vi "2ndStrikerNormalV1.vi"(4 "Impulso de\ntime elapsed":bool=TRUE, 5 "Stop":bool, 6 "atacando ao contrário?":bool=TRUE, 7 "AI Parameters":T1={"GotoKick"={"Dist do cone a frente"=150.0, "attacker farback"=1500.0, "Perto"=300.0, "min dist to kick"=150.0, "kick eps"=0.0, "Time to transition"=0.05}, "Attacker"={"CC chute"=0.09, "CC passe"=0.045, "Kick Force"=100.0, "ball-robot Kick"=200.0, "ball-robot Pass"=0.3, "drible\nAttk"=FALSE}, "Defender"={"D max"=1700.0, "Vel p/ robô av"=1000.0, "Kick Force"=100.0, "D atk-def"=0.0, "D farback"=0.0, "drible\ndef"=FALSE, "drible\ngoalie"=FALSE}, "Timeout"={"Field/v in x"=6.0, "Dist Robots"=300, "Dist up in y"=300}, "Pose Striker"={"dist"=200.0, "Numeric"=-4.0, "dist 2"=200.0, "drible\nstriker"=FALSE}, "Dist Stop"=300.0, "D ball out"=200, "D central gap "=150.0, "T pass"=0.0, "Force ++"=0.0, "range kick"=0.0, "Chute alto"=TRUE, "Marcador novo"=TRUE, "drible"=FALSE, "D drible"=300.0, "Versão Striker"=enum."3", "Defesa"=enum."ManMark", "Marcador"=enum."Marcar Segndo mais perigoso", "Receptor passe"=enum."2nd Striker"} {"D drible" format="%#_13g"; "D central gap" format="%#_13g"; "Dist Stop" format="%#_13g"; "Pose Striker"."Numeric" format="%#_13g"; "Defender"."Kick Force" format="%#_13g"; "Defender"."Vel p/ robô av" format="%#_13g"; "Attacker"."ball-robot Kick" format="%#_13g"; "Attacker"."Kick Force" format="%#_13g"; "Attacker"."CC passe" format="%#_13g"; "Attacker"."CC chute" format="%#_13g"; "GotoKick"."kick eps" format="%#_13g"; "GotoKick"."min dist to kick" format="%#_13g"; "GotoKick"."Perto" format="%#_13g"; "GotoKick"."attacker farback" format="%#_13g"; "GotoKick"."Dist do cone a frente" format="%#_13g"}, 8 "IA Input":T9={"our_robots"=[], "enemy_robots"=[], "balls"=[], "geometry"={"line_width"=0, "field_length"=0, "field_width"=0, "boundary_width"=0, "referee_width"=0, "goal_width"=0, "goal_depth"=0, "goal_wall_width"=0, "center_circle_radius"=0, "defense_radius"=0, "defense_stretch"=0, "free_kick_from_defense_dist"=0, "penalty_spot_from_field_line_dist"=0, "penalty_line_from_spot_dist"=0}, "IA Judge"={"stage"="", "command"="", "our_goalie_id"=0.0, "enemy_goalie_id"=0.0, "command enum"=enum."Halt", "Time"=enum."Azul"}, "Received Timestamp"=timestamp(0 s since 1904-01-01), "Events"={"Touch"=FALSE, "Ball out"=FALSE, "id touch"=0.0, "Ball out of \nVision"=FALSE, "Ball inside \nGoalie area"=FALSE, "Robot not responding"=FALSE, "Robots responding status"=[1.0, 1.0, 1.0, 1.0, 1.0, 1.0], "Enemy Ball \nPossession"=FALSE, "Pass State"=FALSE, "id end of pass"=0.0, "Kick"=FALSE, "Id ini Possession"=0.0, "Ball Possesion"=FALSE, "Id Possesion"=0.0, "Direct Kick"=FALSE, "2nd Strk Ativo"=FALSE}}, 9 "balls":T7[](array[typedef])=[{"x"=-2165.869384765625, "y"=510.4085693359375, "timestamp"=timestamp(2082758857.4639893 s since 1904-01-01), "Vel_x"=0.0, "Vel_y"=0.0, "Pos Bola Est"=[]}], 10 "Field Size in":T8={"line_width"=10, "field_length"=6000, "field_width"=4000, "boundary_width"=250, "referee_width"=425, "goal_width"=700, "goal_depth"=180, "goal_wall_width"=20, "center_circle_radius"=500, "defense_radius"=500, "defense_stretch"=350, "free_kick_from_defense_dist"=700, "penalty_spot_from_field_line_dist"=450, "penalty_line_from_spot_dist"=350}, 11 "Robot in":T2={"id"=5, "function"=enum."Attacker", "x"=-1842.5054931640625, "y"=520.60986328125, "orientation"=-2.7555055618286133, "v_tangent"=0.0, "v_normal"=0.0, "v_ang"=0.0, "kick_x"=0.0, "kick_z"=0.0, "dribble"=FALSE, "Timestamp"=timestamp(2082758857.4639893 s since 1904-01-01), "estimatives"={"est_v_tangent"=0.0, "est_v_normal"=0.0, "est_vx"=0.0, "est_vy"=0.0, "Pos Robot Est"=[]}, "dest_x_kick"=0.0, "dest_y_kick"=0.0, "Gap Coord"=[], "States"=enum."GoToTangent", "Path "=[], "Path  Smooth"=[], "Dest"=[]}) -> (2 "Robot out":T2={"id"=5, "function"=enum."Attacker", "x"=-1842.5054931640625, "y"=520.60986328125, "orientation"=-2.7555055618286133, "v_tangent"=-0.08361641967936218, "v_normal"=-0.20513016702014014, "v_ang"=0.24456003022714357, "kick_x"=0.0, "kick_z"=0.0, "dribble"=FALSE, "Timestamp"=timestamp(2082758857.4639893 s since 1904-01-01), "estimatives"={"est_v_tangent"=0.0, "est_v_normal"=0.0, "est_vx"=0.0, "est_vy"=0.0, "Pos Robot Est"=[]}, "dest_x_kick"=0.0, "dest_y_kick"=0.0, "Gap Coord"=[], "States"=enum."GoToTangent", "Path "=[], "Path  Smooth"=[], "Dest"=[]})   [LabVIEW 2017]
uses:
  Core/AI Robot.ctl
  Functions Enum.ctl
  AttackerStates.ctl
  Path Planning/RRT/PathDests.ctl
  Path Planning/RRT/PathDest.ctl
  Core/AI Input.ctl
  Core/AI Ball.ctl
  Core/Field Size.ctl
  Core/AI Judge.ctl
  Command Enum.ctl
  Util/Events/Events.ctl
  AI Parameters.ctl
panel:
  in  "Wait pass perpendicular?":bool=TRUE
  in  "Marcador sempre":bool
  out "size(s)":i32
  in  "IDattacker":dbl
  in  "Yattacker":dbl
  in  "Xattacker":dbl
  out "States":T4
  out "sentido":dbl
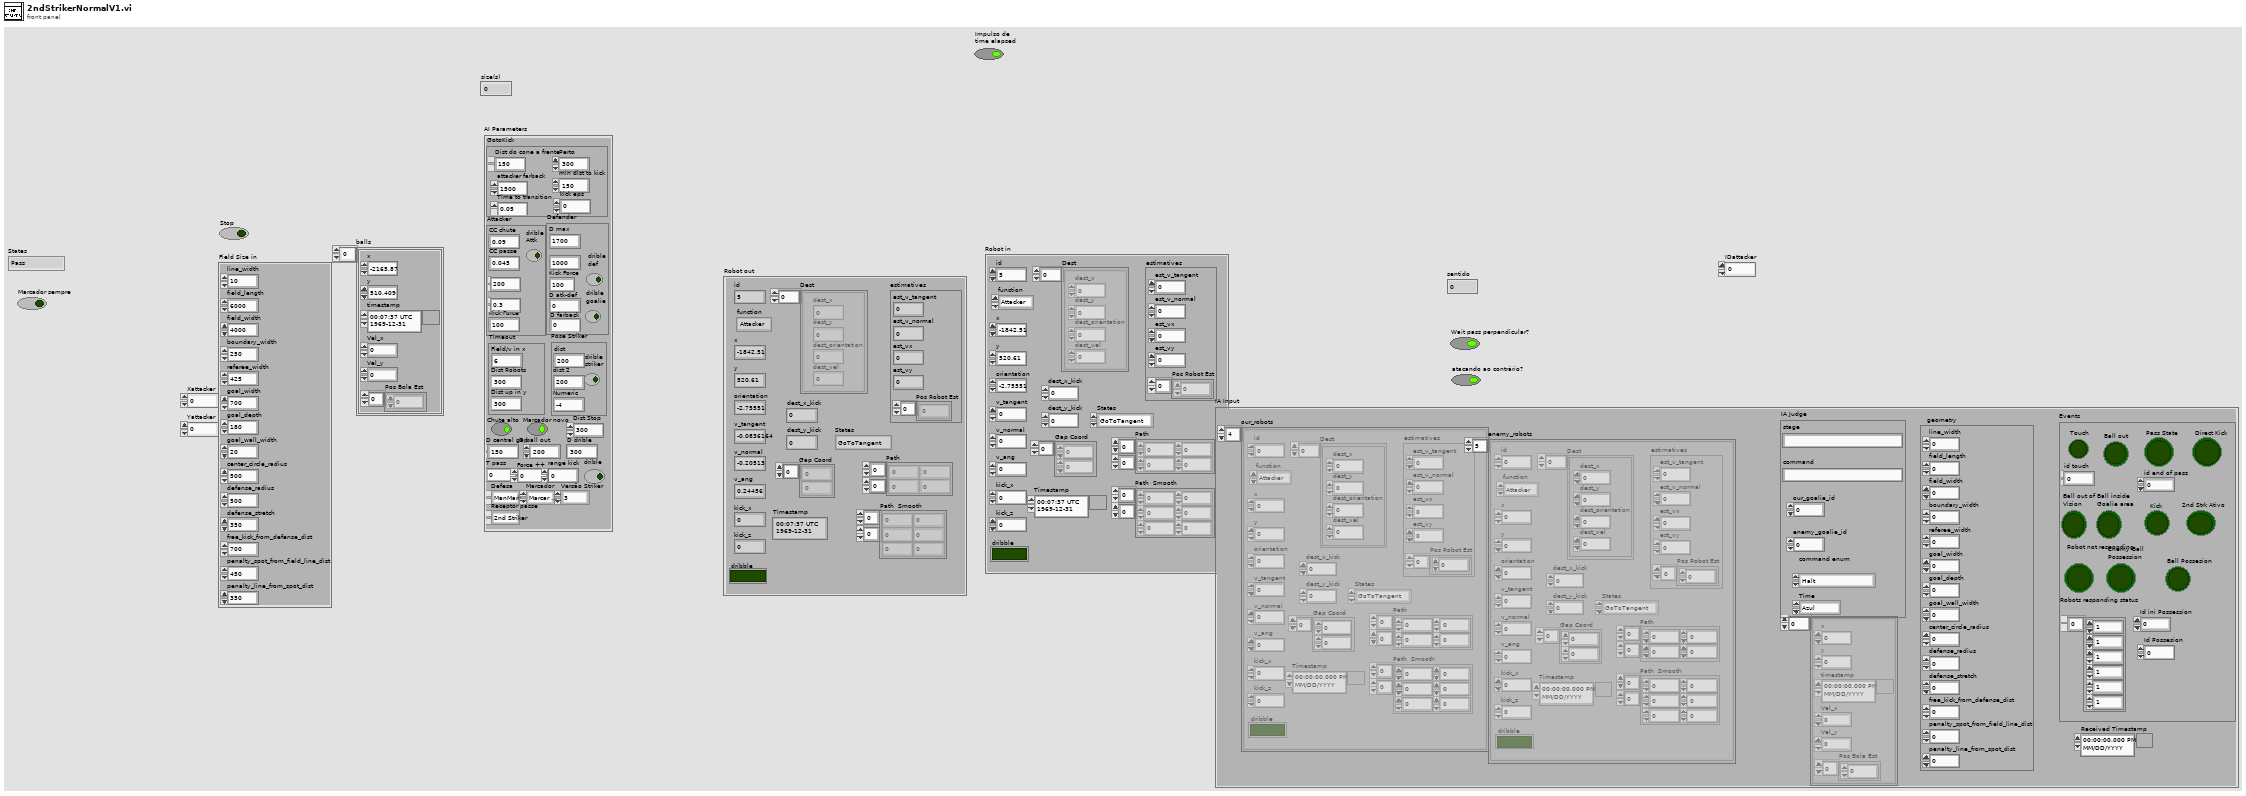
[diagram p1: front panel]
types:
  T1 = typedef "AI Parameters.ctl" = cluster{"GotoKick":cluster{"Dist do cone a frente":dbl, "attacker farback":dbl, "Perto":dbl, "min dist to kick":dbl, "kick eps":dbl, "Time to transition":dbl}, "Attacker":cluster{"CC chute":dbl, "CC passe":dbl, "Kick Force":dbl, "ball-robot Kick":dbl, "ball-robot Pass":dbl, "drible\nAttk":bool}, "Defender":cluster{"D max":dbl, "Vel p/ robô av":dbl, "Kick Force":dbl, "D atk-def":dbl, "D farback":dbl, "drible\ndef":bool, "drible\ngoalie":bool}, "Timeout":cluster{"Field/v in x":dbl, "Dist Robots":u32, "Dist up in y":u32}, "Pose Striker":cluster{"dist":dbl, "Numeric":dbl, "dist 2":dbl, "drible\nstriker":bool}, "Dist Stop":dbl, "D ball out":i32, "D central gap ":dbl, "T pass":dbl, "Force ++":dbl, "range kick":dbl, "Chute alto":bool, "Marcador novo":bool, "drible":bool, "D drible":dbl, "Versão Striker":enum16{"3", "2", "1"}, "Defesa":enum16{"ManMark", "Barreira"}, "Marcador":enum16{"Marcar Segndo mais perigoso", "Marcar o mais perigoso"}, "Receptor passe":enum16{"2nd Striker", "Striker"}}
  T2 = typedef "AI Robot.ctl" = cluster{"id":u32, "function":T3, "x":dbl, "y":dbl, "orientation":dbl, "v_tangent":dbl, "v_normal":dbl, "v_ang":dbl, "kick_x":dbl, "kick_z":dbl, "dribble":bool, "Timestamp":timestamp, "estimatives":cluster{"est_v_tangent":dbl, "est_v_normal":dbl, "est_vx":dbl, "est_vy":dbl, "Pos Robot Est":dbl[]}, "dest_x_kick":dbl, "dest_y_kick":dbl, "Gap Coord":dbl[], "States":T4, "Path ":dbl[][], "Path  Smooth":dbl[][], "Dest":T5}
  T3 = typedef "Functions Enum.ctl" = enum16{"2nd Striker", "Attacker", "Goalie", "Defender", "Striker", "Goto 0", "Dummy", "Kicker", "ZigZag 0", "ZigZag 1", "ZigZag 2", "ZigZag 3", "ZigZag 4", "ZigZag 5", "ZigZag 6", "ZigZag 7", "ZigZag 8", ""}
  T4 = typedef "AttackerStates.ctl" = enum16{"Pass", "GoToTangent", "BallGetting", "GoToKick", ""}
  T5 = typedef "PathDests.ctl" = T6[]
  T6 = typedef "PathDest.ctl" = cluster{"dest_x":dbl, "dest_y":dbl, "dest_orientation":dbl, "dest_vel":dbl}
  T7 = typedef "AI Ball.ctl" = cluster{"x":dbl, "y":dbl, "timestamp":timestamp, "Vel_x":dbl, "Vel_y":dbl, "Pos Bola Est":dbl[]}
  T8 = typedef "Field Size.ctl" = cluster{"line_width":u32, "field_length":u32, "field_width":u32, "boundary_width":u32, "referee_width":u32, "goal_width":u32, "goal_depth":u32, "goal_wall_width":u32, "center_circle_radius":u32, "defense_radius":u32, "defense_stretch":u32, "free_kick_from_defense_dist":u32, "penalty_spot_from_field_line_dist":u32, "penalty_line_from_spot_dist":u32}
  T9 = typedef "AI Input.ctl" = cluster{"our_robots":T2[], "enemy_robots":T2[], "balls":T7[], "geometry":T8, "IA Judge":T10, "Received Timestamp":timestamp, "Events":T12}
  T10 = typedef "AI Judge.ctl" = cluster{"stage":string, "command":string, "our_goalie_id":dbl, "enemy_goalie_id":dbl, "command enum":T11, "Time":enum16{"Azul", "Amarelo"}}
  T11 = typedef "Command Enum.ctl" = enum16{"Halt", "Stop", "Force Start", "PKA Normal Start", "Prepare Kickoff Ally", "PKE Normal Start", "Prepare Kickoff Enemy", "Prepare Penalty Ally", "PPA Normal Start", "Prepare Penalty Enemy", "PPE Normal Start", "Direct Free Enemy", "Direct Free Ally", "Indirect Free Enemy", "Indirect Free Ally", "Timeout Enemy", "Timeout Ally", "Goal Enemy", "Goal Ally", "Ball Placement Enemy", "Ball Placement Ally", "Normal Half Time", "Extra Time Break", "Extra Half Time", "None", "Post Game"}
  T12 = typedef "Events.ctl" = cluster{"Touch":bool, "Ball out":bool, "id touch":dbl, "Ball out of \nVision":bool, "Ball inside \nGoalie area":bool, "Robot not responding":bool, "Robots responding status":dbl[], "Enemy Ball \nPossession":bool, "Pass State":bool, "id end of pass":dbl, "Kick":bool, "Id ini Possession":dbl, "Ball Possesion":bool, "Id Possesion":dbl, "Direct Kick":bool, "2nd Strk Ativo":bool}
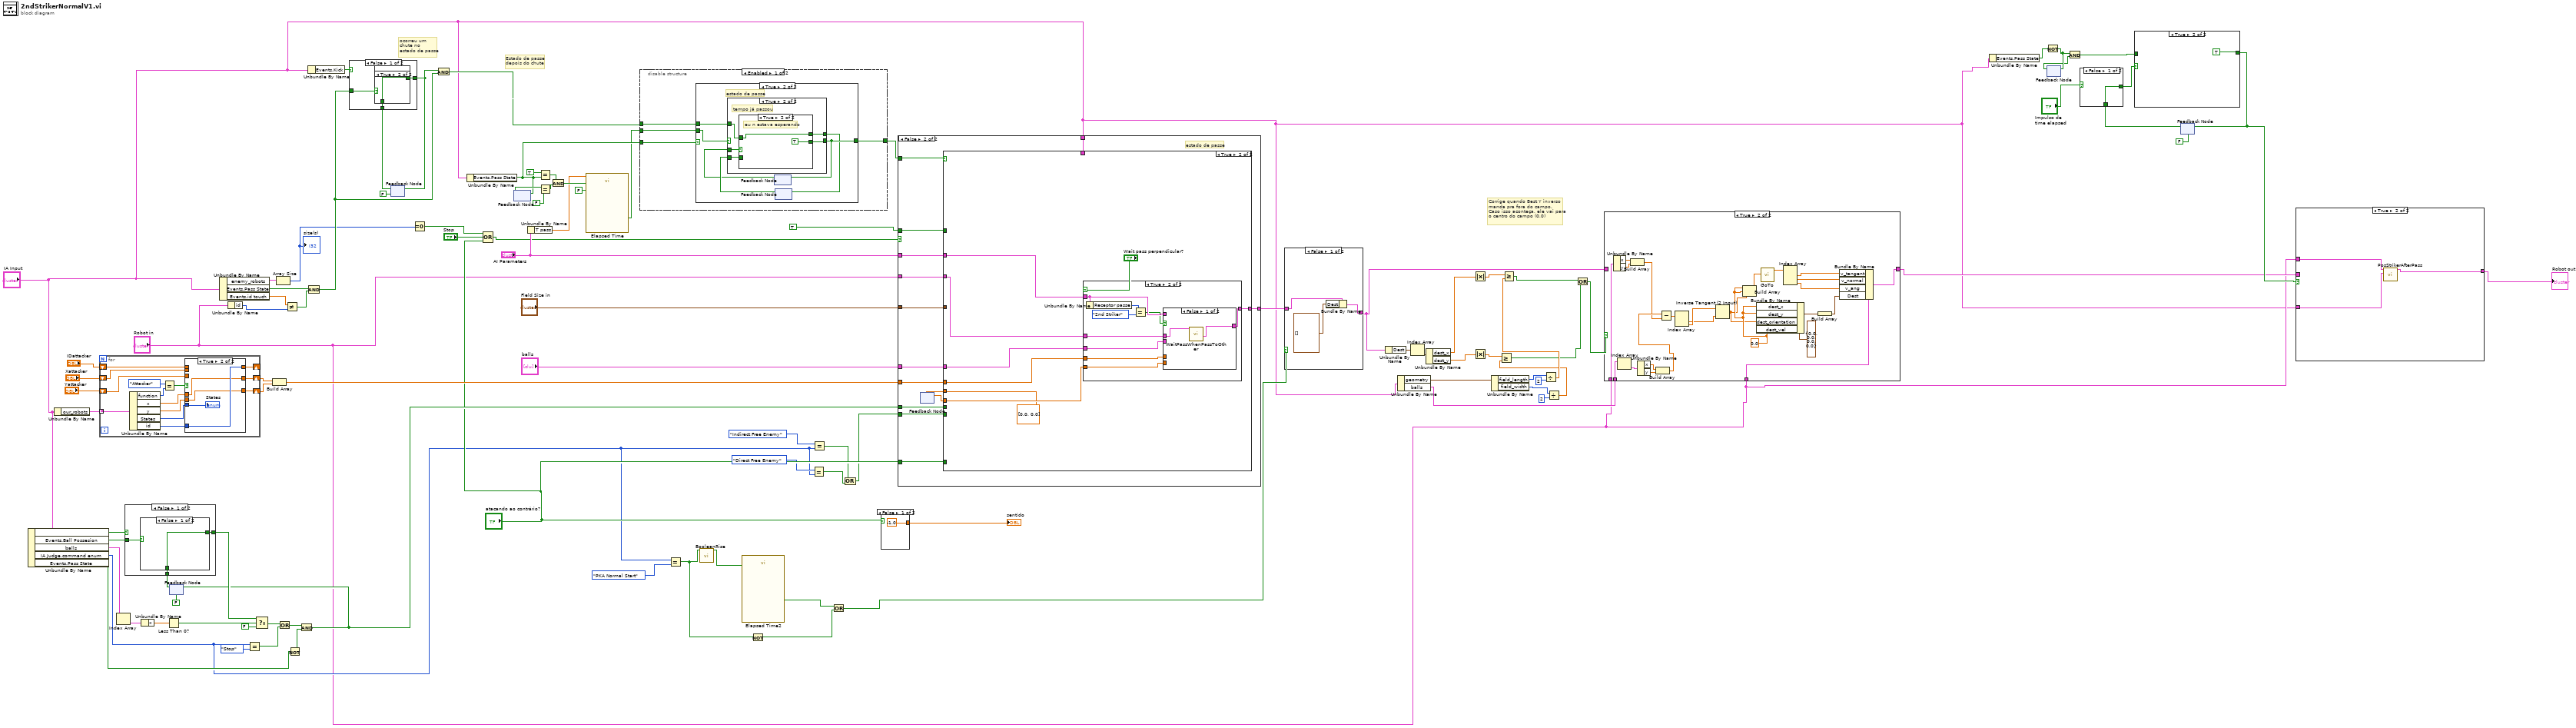
[diagram p0: block diagram]
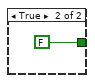
[diagram p2: hidden frame]
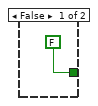
[diagram p7: hidden frame]
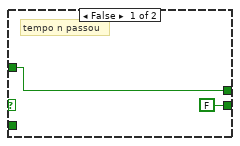
[diagram p8: hidden frame]
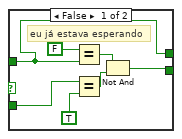
[diagram p9: hidden frame]
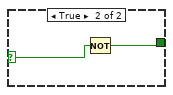
[diagram p11: hidden frame]
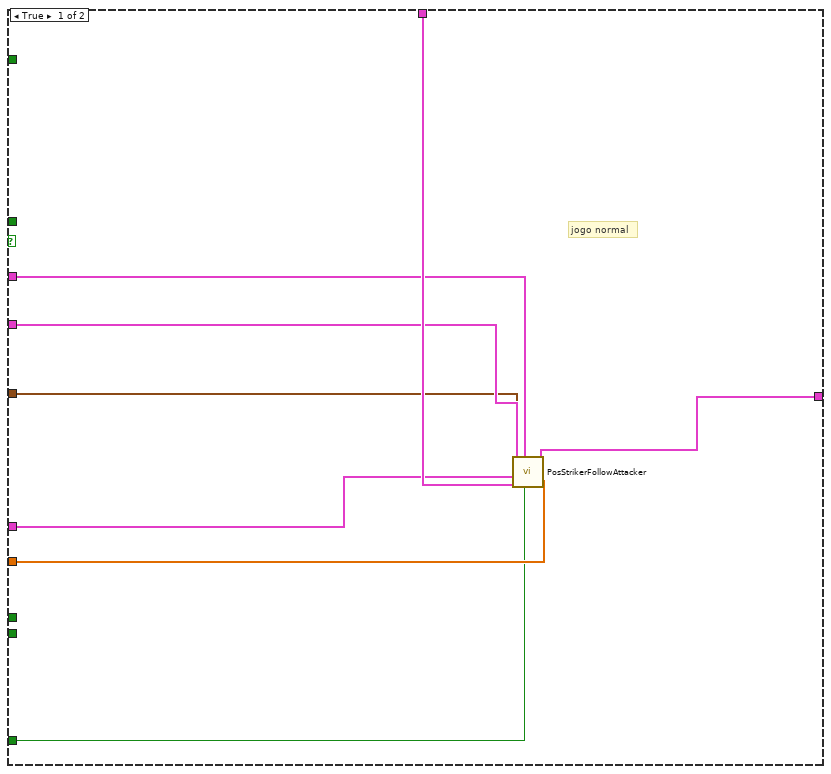
[diagram p13: hidden frame]
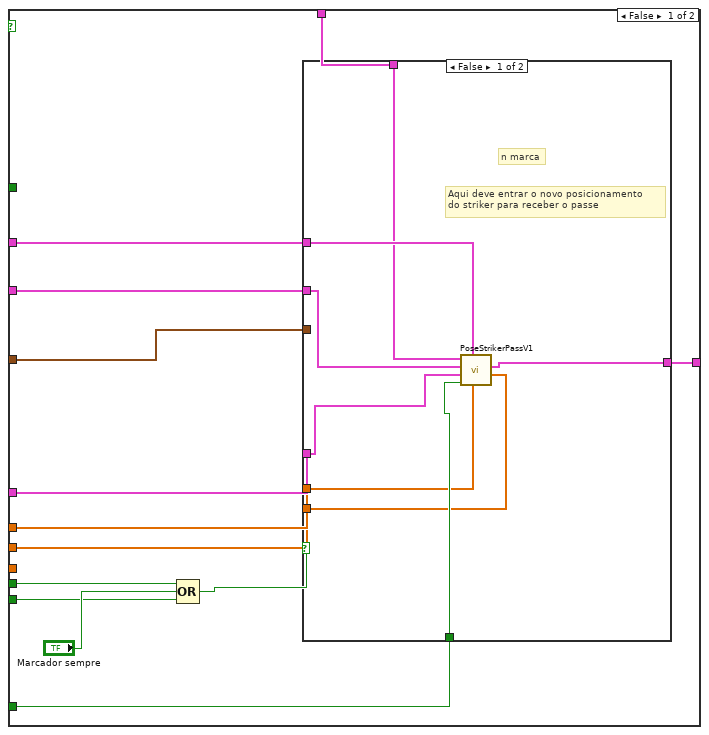
[diagram p14: hidden frame]
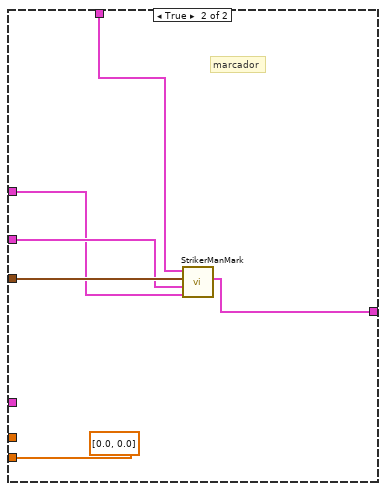
[diagram p15: hidden frame]
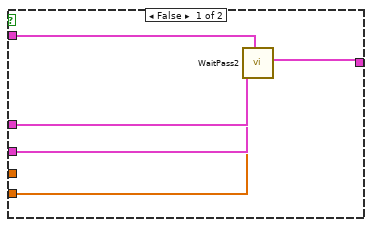
[diagram p16: hidden frame]
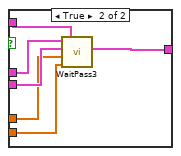
[diagram p17: hidden frame]
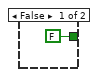
[diagram p19: hidden frame]
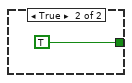
[diagram p20: hidden frame]
diagram:
  # "Corrige quando Best Y inverso\nmanda pra fora do campo.\nCaso isso aconteça, ele vai para\no centro do campo (0,0)"
  # "ocorreu um \nchute no\nestado de passe"
  # "Estado de passe\ndepois do chute"
  n1 = Unbundle By Name("IA Input") -> ("Events.Enemy Ball \nPossession"=w79:bool, "Events.Ball Possesion"=w78:bool, "balls"=w76:T7[], "IA Judge.command enum"=w39:T11, "Events.Pass State"=w66:bool)
  n2 = Unbundle By Name("IA Input") -> ("our_robots"=w94:T2[])
  n3 = for {
    tunnel: w94 -> [w109] mode=indexing
    shift-right: [w105] -> w90
    shift-left: "Xattacker" -> [w103]
    shift-right: [w104] -> w89
    shift-left: "Yattacker" -> [w102]
    shift-right: [w106] -> _
    shift-left: "IDattacker" -> [w101]
    n4 = Unbundle By Name(w109) -> ("function"=w114:T3, "x"=w111:dbl, "y"=w110:dbl, "States"=w108:T4, "id"=w107:u32)
    n5 = Equal?(x=Functions_Enum."Attacker", y=w114) -> (x = y?=w112:bool)
    n6 = case shown="True" w112 {
      tunnel: w111 -> [_ w119]
      tunnel: w110 -> [_ w118]
      tunnel: w108 -> [_ w121]
      tunnel: w107 -> [_ w120]
      tunnel: [w115 w120] -> w106
      tunnel: [w117 w119] -> w105
      tunnel: [w116 w118] -> w104
      tunnel: w103 -> [w117 _]
      tunnel: w102 -> [w116 _]
      tunnel: w101 -> [w115 _]
      frame False {
      }
      frame True {
        "States" <- w121
      }
    }
  }
  n7 = Index Array(array=w76) -> (element=w75:T7)  [unwired: 1 in]
  n8 = Unbundle By Name(w75) -> ("x"=w74:dbl)
  n9 = Less Than 0?(x=w74) -> (x < 0?=w73:bool)
  n10 = feedback #1(FALSE) -> (w77:bool)
  n11 = case shown="False" w79 {
    selector: w79 -> [_ w128]
    tunnel: [w123 w128] -> w72
    tunnel: w78 -> [w124 _]
    tunnel: w77 -> [w122 _]
    frame False {
      n12 = case shown="False" w124 {
        selector: w124 -> [_ w126]
        tunnel: [w125 w127] -> w123
        tunnel: w122 -> [w125 _]
        frame False {
        }
        frame True {
          n13 = Not(x=w126) -> (.not. x?=w127:bool)
        }
      }
    }
    frame True {
    }
  }
  n14 = Unbundle By Name("IA Input") -> ("enemy_robots"=w52:T2[], "Events.Pass State"=w95:bool, "Events.id touch"=w84:dbl)
  n15 = Unbundle By Name("Robot in") -> ("id"=w83:u32)
  n16 = Equal?(x=w39, y=Command_Enum."Stop") -> (x = y?=w69:bool)
  n17 = Select(t=w72, s=w73, f=FALSE) -> (s? t:f=w70:bool)
  n18 = Build Array(w90, w89) -> (w88:dbl[])
  n19 = Array Size(array=w52) -> (size(s)=w50:i32)
  "size(s)" <- w50
  n20 = Or(x=w70, y=w69) -> (x .or. y?=w67:bool)
  n21 = Not Equal?(x=w84, y=w83) -> (x != y?=w85:bool)
  n22 = Not(x=w66) -> (.not. x?=w65:bool)
  n23 = And(x=w67, y=w65) -> (x .and. y?=w64:bool)
  n24 = feedback-in #1(w64) -> ()
  n25 = Unbundle By Name("IA Input") -> ("Events.Kick"=w99:bool)
  n26 = Compound Arithmetic op=AND(w95, w85) -> (w86:bool)
  n27 = feedback #2(FALSE) -> (w97:bool)
  n28 = case shown="False" w99 {
    tunnel: [w130 TRUE] -> w98
    tunnel: w97 -> [w129 _]
    tunnel: w86 -> [w131 _]
    frame False {
      n29 = case shown="True" w131 {
        tunnel: [FALSE w133] -> w130
        tunnel: w129 -> [_ w133]
        frame False {
        }
        frame True {
        }
      }
    }
    frame True {
    }
  }
  n30 = feedback-in #2(w98) -> ()
  n31 = Equal To 0?(x=w50) -> (x = 0?=w51:bool)
  n32 = And(x=w98, y=w86) -> (x .and. y?=w55:bool)
  n33 = Unbundle By Name("IA Input") -> ("Events.Pass State"=w54:bool)
  n34 = Compound Arithmetic op=OR(w51, "Stop", "atacando ao contrário?") -> (w47:bool)
  n35 = feedback #3() -> (w63:bool)  [unwired: 1 in]
  n36 = feedback-in #3(w54) -> ()
  n37 = Unbundle By Name("AI Parameters") -> ("T pass"=w48:dbl)
  n38 = Equal?(x=TRUE, y=w54) -> (x = y?=w59:bool)
  n39 = Equal?(x=w63, y=FALSE) -> (x = y?=w60:bool)
  n40 = And(x=w59, y=w60) -> (x .and. y?=w58:bool)
  n41 = call "Elapsed Time"("Time Target (s)"=w48, "Reset"=w58, "Auto Reset"=FALSE) -> ("Time has Elapsed"=w53:bool)  [unwired: 9 in, 7 out]
  n42 = disable-structure shown="Enabled" {
    disable-tunnel: w53 -> [w136 _]
    disable-tunnel: [w138 w162] -> w56
    disable-tunnel: w55 -> [w137 w162]
    disable-tunnel: w54 -> [w135 _]
    frame Enabled {
      n43 = case shown="True" w135 {
        tunnel: [FALSE w145] -> w138
        tunnel: w137 -> [_ w144]
        tunnel: w136 -> [_ w141]
        frame False {
        }
        frame True {
          # "estado de passe"
          n44 = feedback #4() -> (w140:bool)  [unwired: 1 in]
          n45 = feedback #5() -> (w142:bool)  [unwired: 1 in]
          n46 = case shown="True" w141 {
            tunnel: [FALSE w151] -> w145
            tunnel: w144 -> [w146 w150]
            tunnel: [w146 w148] -> w143
            tunnel: w142 -> [_ w149]
            tunnel: w140 -> [_ w152]
            frame False {
              # "tempo n passou"
            }
            frame True {
              # "tempo já passou"
              n47 = case shown="True" w152 {
                tunnel: [w154 TRUE] -> w151
                tunnel: w150 -> [w153 w160]
                tunnel: w149 -> [w155 _]
                tunnel: [w153 w160] -> w148
                frame False {
                  # "eu já estava esperando"
                  n48 = Equal?(x=FALSE, y=w153) -> (x = y?=w156:bool)
                  n49 = Equal?(x=w155, y=TRUE) -> (x = y?=w157:bool)
                  n50 = Not And(1:w157, 2:w156) -> (0:w154:bool)
                }
                frame True {
                  # "eu n estava esperando"
                }
              }
            }
          }
          n51 = feedback-in #4(w145) -> ()
          n52 = feedback-in #5(w143) -> ()
        }
      }
    }
    frame Disabled {
    }
  }
  n53 = Equal?(x=w39, y=Command_Enum."PKA Normal Start") -> (x = y?=w35:bool)
  n54 = call "BooleanRise.vi"("Test Mode On"=w35) -> ("Boolean"=w37:bool)  [unwired: 10 in]
  n55 = call "Elapsed Time2"("Reset"=w37) -> ("Time has Elapsed"=w33:bool)  [unwired: 11 in, 7 out]
  n56 = Not(x=w35) -> (.not. x?=w34:bool)
  n57 = Equal?(x=Command_Enum."Direct Free Enemy", y=w39) -> (x = y?=w42:bool)
  n58 = Equal?(x=Command_Enum."Indirect Free Enemy", y=w39) -> (x = y?=w41:bool)
  n59 = Or(x=w33, y=w34) -> (x .or. y?=w32:bool)
  n60 = Compound Arithmetic op=OR(w41, w42) -> (w40:bool)
  n61 = case shown="False" "atacando ao contrário?" {
    tunnel: [-1.0 1.0] -> w100
    frame False {
    }
    frame True {
    }
  }
  "sentido" <- w100
  n62 = case shown="False" w47 {
    tunnel: w56 -> [_ w178]
    tunnel: TRUE -> [_ w179]
    tunnel: "Robot in" -> [w171 w186]
    tunnel: w88 -> [w168 w185]
    tunnel: "atacando ao contrário?" -> [w167 w184]
    tunnel: "Field Size in" -> [w170 w183]
    tunnel: "balls" -> [w169 w182]
    tunnel: "IA Input" -> [w172 w181]
    tunnel: [w166 w180] -> w36
    tunnel: "AI Parameters" -> [w165 w177]
    tunnel: w64 -> [_ w176]
    tunnel: w40 -> [_ w173]
    frame True {
      # "jogo normal"
      n63 = call "PosStrikerFollowAttacker.vi"("Pos Attacker"=w168, "atacando ao contrário?"=w167, "AI Parameters"=w165, "IA Input"=w172, "balls"=w169, "Field Size in"=w170, "Robot in"=w171) -> ("Robot out"=w166:T2)  [unwired: 4 in]
    }
    frame False {
      # "estado de passe"
      n64 = feedback #6() -> (w174:dbl[])  [unwired: 1 in]
      n65 = case shown="True" w178 {
        tunnel: w179 -> [_ _]
        tunnel: w186 -> [w198 w221]
        tunnel: w185 -> [w193 w214]
        tunnel: [w195 w220] -> w180
        tunnel: w184 -> [w199 _]
        tunnel: w183 -> [w192 _]
        tunnel: w182 -> [w197 w219]
        tunnel: w181 -> [w196 _]
        tunnel: w177 -> [w194 w215]
        tunnel: w176 -> [w191 _]
        tunnel: [w188 dbl[] [0.0, 0.0] ("FinalPosition")] -> w175
        tunnel: w174 -> [_ w218]
        tunnel: w173 -> [w187 _]
        frame False {
          n66 = Compound Arithmetic op=OR(w191, "Marcador sempre", w187) -> (w190:bool)
          n67 = case shown="False" w190 {
            tunnel: w199 -> [w203 _]
            tunnel: w198 -> [w205 w212]
            tunnel: w197 -> [w202 _]
            tunnel: w196 -> [w204 w210]
            tunnel: [w207 w211] -> w195
            tunnel: w194 -> [w206 w209]
            tunnel: w193 -> [w201 _]
            tunnel: w192 -> [_ w213]
            tunnel: [w200 dbl[] [0.0, 0.0] ("FinalPosition")] -> w188
            frame False {
              # "n marca"
              # "Aqui deve entrar o novo posicionamento\ndo striker para receber o passe"
              n68 = call "PoseStrikerPassV1.vi"("Array"=w201, "AI Parameters"=w206, "atacando ao contrário?"=w203, "balls"=w202, "Robot in"=w205, "IA Input"=w204) -> ("FinalPosition"=w200:dbl[], "Robot out"=w207:T2)  [unwired: 4 in]
            }
            frame True {
              # "marcador"
              n69 = call "StrikerManMark.vi"("AI Parameters"=w209, "Robot in"=w212, "Field Size in"=w213, "IA Input"=w210) -> ("Robot out"=w211:T2)  [unwired: 6 in, 1 out]
            }
          }
        }
        frame True {
          n70 = case shown="True" "Wait pass perpendicular?" {
            tunnel: w221 -> [w225 w231]
            tunnel: [w226 w235] -> w220
            tunnel: w219 -> [w224 w234]
            tunnel: w218 -> [w223 w232]
            tunnel: w215 -> [w222 w230]
            tunnel: w214 -> [_ w233]
            frame False {
              n71 = call "WaitPass2.vi"("AI Parameters"=w222, "Best Y Inverso"=w223, "balls"=w224, "Robot in"=w225) -> ("Robot out"=w226:T2)  [unwired: 7 in]
            }
            frame True {
              n72 = Unbundle By Name(w230) -> ("Receptor passe"=w229:enum16{"2nd Striker", "Striker"})
              n73 = Equal?(x=w229, y=enum16{"2nd Striker", "Striker"}."2nd Striker") -> (x = y?=w227:bool)
              n74 = case shown="False" w227 {
                tunnel: [w237 w243] -> w235
                tunnel: w234 -> [_ w242]
                tunnel: w230 -> [_ w241]
                tunnel: w233 -> [_ w240]
                tunnel: w232 -> [_ w239]
                tunnel: w231 -> [w236 w238]
                frame False {
                  n75 = call "WaitPassWhenPassToOther.vi"("Robot in"=w236) -> ("Robot out"=w237:T2)  [unwired: 10 in]
                }
                frame True {
                  n76 = call "WaitPass3.vi"("AI Parameters"=w241, "Best Y Inverso"=w239, "Target"=w240, "balls"=w242, "Robot in"=w238) -> ("Robot out"=w243:T2)  [unwired: 6 in]
                }
              }
            }
          }
        }
      }
      n77 = feedback-in #6(w175) -> ()
    }
  }
  n78 = case shown="False" w32 {
    tunnel: [w245 w247] -> w15
    tunnel: w36 -> [w246 w247]
    frame False {
      n79 = Bundle By Name(cluster=w246, "Dest"=T5 []) -> (w245:T2)
    }
    frame True {
    }
  }
  n80 = Unbundle By Name(w15) -> ("Dest"=w19:T5)
  n81 = Unbundle By Name("IA Input") -> ("geometry"=w31:T8, "balls"=w14:T7[])
  n82 = Index Array(array=w19) -> (element=w18:T6)  [unwired: 1 in]
  n83 = Unbundle By Name(w18) -> ("dest_x"=w17:dbl, "dest_y"=w16:dbl)
  n84 = Absolute Value(x=w17) -> (abs(x)=w26:dbl)
  n85 = Absolute Value(x=w16) -> (abs(x)=w24:dbl)
  n86 = Unbundle By Name(w31) -> ("field_length"=w30:u32, "field_width"=w27:u32)
  n87 = Divide(x=w30, y=2) -> (x/y=w25:dbl)
  n88 = Greater Or Equal?(x=w26, y=w25) -> (x >= y?=w22:bool)
  n89 = Divide(x=w27, y=u32 2) -> (x/y=w23:dbl)
  n90 = Greater Or Equal?(x=w24, y=w23) -> (x >= y?=w21:bool)
  n91 = Or(x=w22, y=w21) -> (x .or. y?=w20:bool)
  n92 = case shown="True" w20 {
    tunnel: [w248 w269] -> w4
    tunnel: w15 -> [w248 _]
    tunnel: "Robot in" -> [_ w268]
    tunnel: w14 -> [_ w262]
    tunnel: "Robot in" -> [_ w258]
    frame False {
    }
    frame True {
      w252 = 0.0 ("dest_vel")
      n93 = Unbundle By Name(w258) -> ("x"=w257:dbl, "y"=w256:dbl)
      n94 = Index Array(array=w262) -> (element=w261:T7)  [unwired: 1 in]
      n95 = Build Array(w257, w256) -> (w249:dbl[])
      n96 = Unbundle By Name(w261) -> ("x"=w260:dbl, "y"=w259:dbl)
      n97 = Build Array(w260, w259) -> (w250:dbl[])
      n98 = Subtract(x=w250, y=w249) -> (x-y=w255:dbl[])
      n99 = Index Array(array=w255) -> (element #1=w253:dbl, element #2=w254:dbl)  [unwired: 2 in]
      n100 = Inverse Tangent (2 Input)(1:w253, 2:w254) -> (0:w251:dbl)
      n101 = Build Array(w252, w252, w251) -> (w263:dbl[])
      n102 = Bundle By Name(cluster=T6 {"dest_x"=0.0, "dest_y"=0.0, "dest_orientation"=0.0, "dest_vel"=0.0} ("Dest"), "dest_x"=w252, "dest_y"=w252, "dest_orientation"=w251, "dest_vel"=w252) -> (w271:T6)
      n103 = call "GoTo.vi"("Target"=w263) -> ("Output\nVelocity"=w267:dbl[])  [unwired: 9 in, 1 out]
      n104 = Index Array(array=w267) -> (element #1=w266:dbl, element #2=w264:dbl, element #3=w265:dbl)  [unwired: 3 in]
      n105 = Build Array(w271) -> (w270:T6[])
      n106 = Bundle By Name(cluster=w268, "v_tangent"=w266, "v_normal"=w264, "v_ang"=w265, "Dest"=w270) -> (w269:T2)
    }
  }
  n107 = Unbundle By Name("IA Input") -> ("Events.Pass State"=w13:bool)
  n108 = Not(x=w13) -> (.not. x?=w12:bool)
  n109 = feedback #7() -> (w11:bool)  [unwired: 1 in]
  n110 = feedback-in #7(w12) -> ()
  n111 = And(x=w12, y=w11) -> (x .and. y?=w10:bool)
  n112 = feedback #8(FALSE) -> (w6:bool)
  n113 = case shown="False" "Impulso de\ntime elapsed" {
    tunnel: [w273 FALSE] -> w7
    tunnel: w6 -> [w273 _]
    frame False {
    }
    frame True {
    }
  }
  n114 = case shown="True" w7 {
    tunnel: [w275 TRUE] -> w5
    tunnel: w10 -> [w275 _]
    frame False {
    }
    frame True {
    }
  }
  n115 = feedback-in #8(w5) -> ()
  n116 = case shown="True" w5 {
    tunnel: [w277 w280] -> w2
    tunnel: w4 -> [w277 _]
    tunnel: "IA Input" -> [_ w279]
    tunnel: "Robot in" -> [_ w278]
    frame False {
    }
    frame True {
      n117 = call "PosStrikerAfterPass.vi"("IA Input"=w279, "Robot in"=w278) -> ("Robot out"=w280:T2)  [unwired: 9 in]
    }
  }
  "Robot out" <- w2
